vi "2014 Target Detection.vi"() -> (0 "Target Info":T6(array[cluster]))   [LabVIEW 2013]
uses:
  <vilib>/Rock Robotics/WPI/Camera/WPI_CameraSettings Read MJPG.ctl
  <vilib>/Rock Robotics/WPI/Camera/WPI_CameraImageSize.ctl
  TargetType.ctl
  <vilib>/vision/NI_Vision_Development_Module.lvlib
panel:
  out "Angle from Robot (deg)":dbl
  out "Polar Plot":picture
  in  "Instructions:":string="Images:\nUse the tab immediately below to choose the image source. Update the camera settings or the image directory so that you have images or video to test with.\n\nCalibration:\nYou can update Color Component ranges directly, or by clicking and drawing a line on the colored strip in the Image control. The Std Dev multipliers and where the strip is drawn determine the calibration values.\n\nUse Debugging tab to view the result of the color range threshold .\n\nArea Size LImit is used to ignore objects too small or far away to care about.\n\nThe Details tab contains score details for each target and subObject.\n\nCamera Type is used to select lens angles for distance calculation.\n\nVertical strips with no adjacent horizontal strip are identified as \"not hot\" and marked in blue.\nThe numeric scores indicate represent aspect ratio and rectangularity.\n\nWhen both strips are near enough, the pair is identified as \"hot\" and marked in green. Scores\nindicate the left, right, ratio of widths, and vertical positioning.\n\nAny score that falls below cutoff is drawn in red and bounding box is drawn in red."
  in  "Std Devs":cluster{"Hue":dbl, "Sat":dbl, "Val":dbl}={"Hue"=4.0, "Sat"=6.0, "Val"=4.0}
  in  "Area Size Limit %":dbl=0.06 format="%#_13g"
  in  "Camera Type":enum16{"206", "1011", "1013"}(ring)=enum."1013"
  out "loop time ms":u32
  in  "Score Cutoff":dbl(slide)=54.248366013071895 scale=0.0..100.0
  in  "Color Components":T1={"Hue"={80.66666412353516, 112.66666412353516}, "Sat"={0.0, 255.0}, "Val"={102.97300720214844, 167.49366760253906}} {"Val" scale=0.0..255.0; "Sat" scale=0.0..255.0; "Hue" scale=0.0..255.0 scale format="%#_3g"}
  out "Error":bool
  in  "Image Source":enum32{"Files", "Camera"}(tab)=enum."Camera"
  in  "List of image files":i32(listbox)
  in  "Image Directory":path=path "2014 Pseudo-Target/2014 Pseudo-Target Active"
  in  "Camera Settings":T2={"fps"=15, "compression"=5, "Image Size"=enum."640x480"}
  in  "Camera IP":string="10.15.10.11"
  in  "Tabbed Info":enum32{"Debugging", "Details"}(tab)
  out "Mask":T4(plugin-control)
  out "Image":T4(plugin-control)
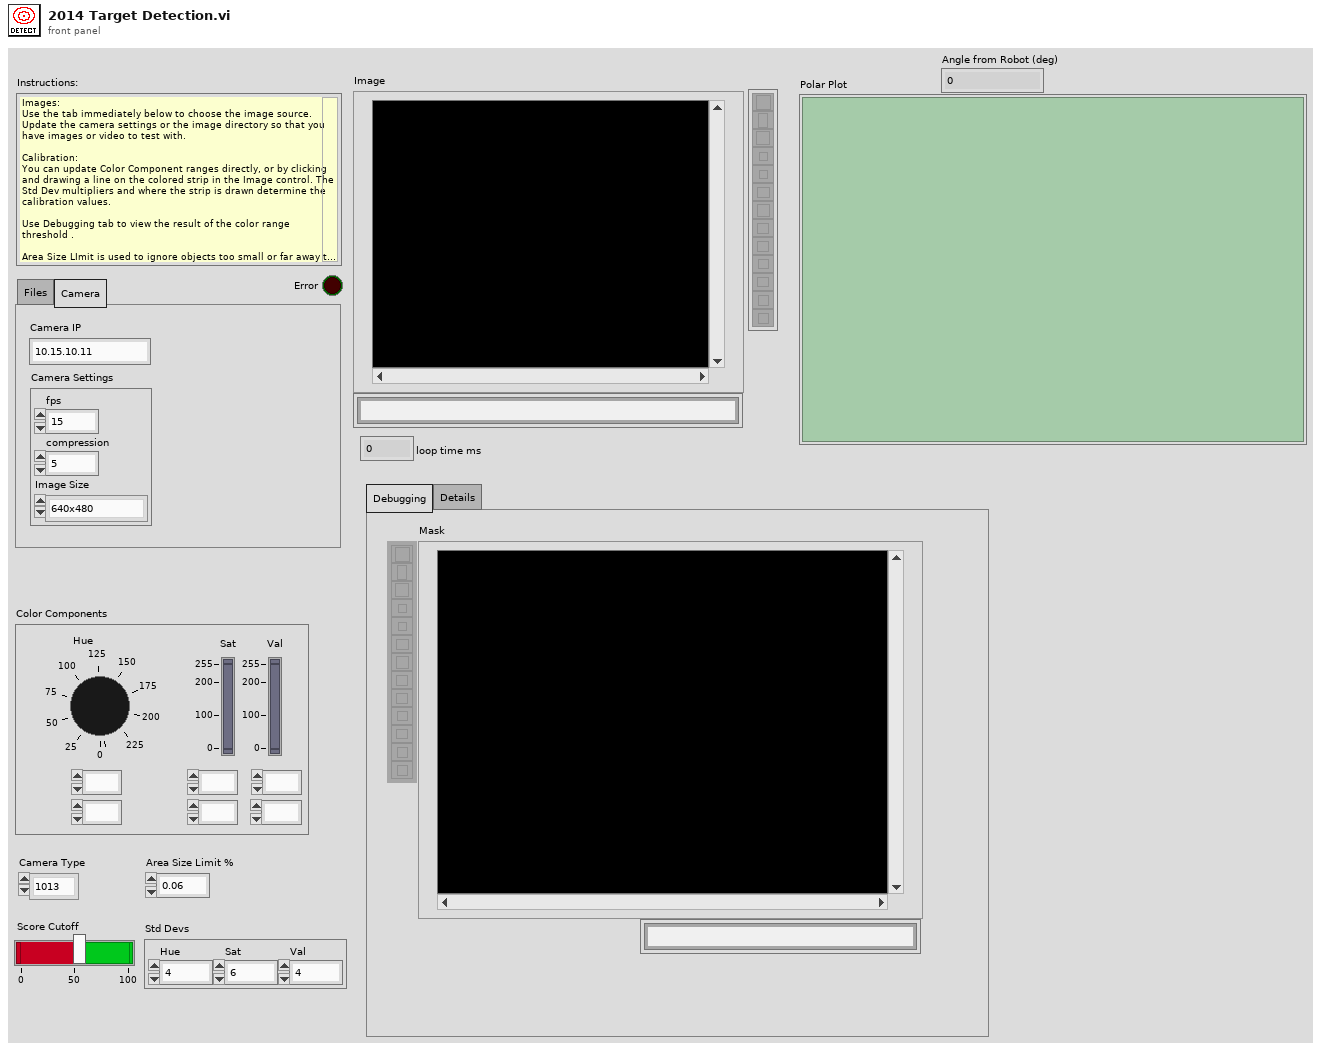
[diagram p1: front panel]
types:
  T1 = cluster{"Hue":cluster{dbl, dbl}, "Sat":cluster{dbl, dbl}, "Val":cluster{dbl, dbl}}
  T2 = typedef "WPI_CameraSettings Read MJPG.ctl" = cluster{"fps":i32, "compression":i32, "Image Size":T3}
  T3 = typedef "WPI_CameraImageSize.ctl" = enum16{"640x480", "320x240", "160x120"}
  T4 = typedef "IMAQ Image.ctl" = refnum<image>
  T5 = typedef "TargetType.ctl" = enum16{"Not Hot", "Hot"}
  T6 = cluster{"Scores":cluster{"Total":dbl, "Left":dbl, "Right":dbl, "Ratio":dbl, "Vertical":dbl, "index":i32, "State":T5}, "Verticals":cluster{"Horizontal?":bool, "Aspect Score":dbl, "Rect Score":dbl, cluster{"Left":dbl, "Top":dbl, "Right":dbl, "Bottom":dbl}, "Equiv H":dbl, "Equiv V":dbl}, "Horizontals":cluster{"Horizontal?":bool, "Aspect Score":dbl, "Rect Score":dbl, cluster{"Left":dbl, "Top":dbl, "Right":dbl, "Bottom":dbl}, "Equiv H":dbl, "Equiv V":dbl}, "Distance ft":dbl, "Center":cluster{"X":dbl, "Y":dbl}}[]
  T7 = typedef "Image Type" = u32
  T8 = cluster{"Horizontal":bool, "Aspect Score":dbl, "Rect Score":dbl, cluster{"Left":dbl, "Top":dbl, "Right":dbl, "Bottom":dbl}, "Equiv H":dbl, "Equiv V":dbl}[]
  T9 = cluster{cluster{dbl, dbl}, cluster{dbl, dbl}, cluster{dbl, dbl}}
  T10 = cluster{"Scores":cluster{"Total":dbl, "Left":dbl, "Right":dbl, "Ratio":dbl, "Vertical":dbl, "index":i32, "State":T5}, "Verticals":cluster{"Horizontal?":bool, "Aspect Score":dbl, "Rect Score":dbl, cluster{"Left":dbl, "Top":dbl, "Right":dbl, "Bottom":dbl}, "Equiv H":dbl, "Equiv V":dbl}, "Horizontals":cluster{"Horizontal?":bool, "Aspect Score":dbl, "Rect Score":dbl, cluster{"Left":dbl, "Top":dbl, "Right":dbl, "Bottom":dbl}, "Equiv H":dbl, "Equiv V":dbl}, "Validated":bool}[]
  T11 = cluster{"Scores":cluster{"Total":dbl, "Left":dbl, "Right":dbl, "Ratio":dbl, "Vertical":dbl, "index":i32, "State":T5}, "Verticals":cluster{"Horizontal?":bool, "Aspect Score":dbl, "Rect Score":dbl, cluster{"Left":dbl, "Top":dbl, "Right":dbl, "Bottom":dbl}, "Equiv H":dbl, "Equiv V":dbl}, "Horizontals":cluster{"Horizontal?":bool, "Aspect Score":dbl, "Rect Score":dbl, cluster{"Left":dbl, "Top":dbl, "Right":dbl, "Bottom":dbl}, "Equiv H":dbl, "Equiv V":dbl}, "Distance (ft)":dbl, "Target Center (-1 to 1)":cluster{"X":dbl, "Y":dbl}}[]
  T12 = cluster{"Scores":cluster{"Total":dbl, "Left":dbl, "Right":dbl, "Ratio":dbl, "Vertical":dbl, "index":i32, "State":T5}, "Verticals":cluster{"Horizontal?":bool, "Aspect Score":dbl, "Rect Score":dbl, cluster{"Left":dbl, "Top":dbl, "Right":dbl, "Bottom":dbl}, "Equiv H":dbl, "Equiv V":dbl}, "Horizontals":cluster{"Horizontal?":bool, "Aspect Score":dbl, "Rect Score":dbl, cluster{"Left":dbl, "Top":dbl, "Right":dbl, "Bottom":dbl}, "Equiv H":dbl, "Equiv V":dbl}, "Distance (ft)":dbl, "Target Center (-1 to 1)":cluster{"X":dbl, "Y":dbl}}
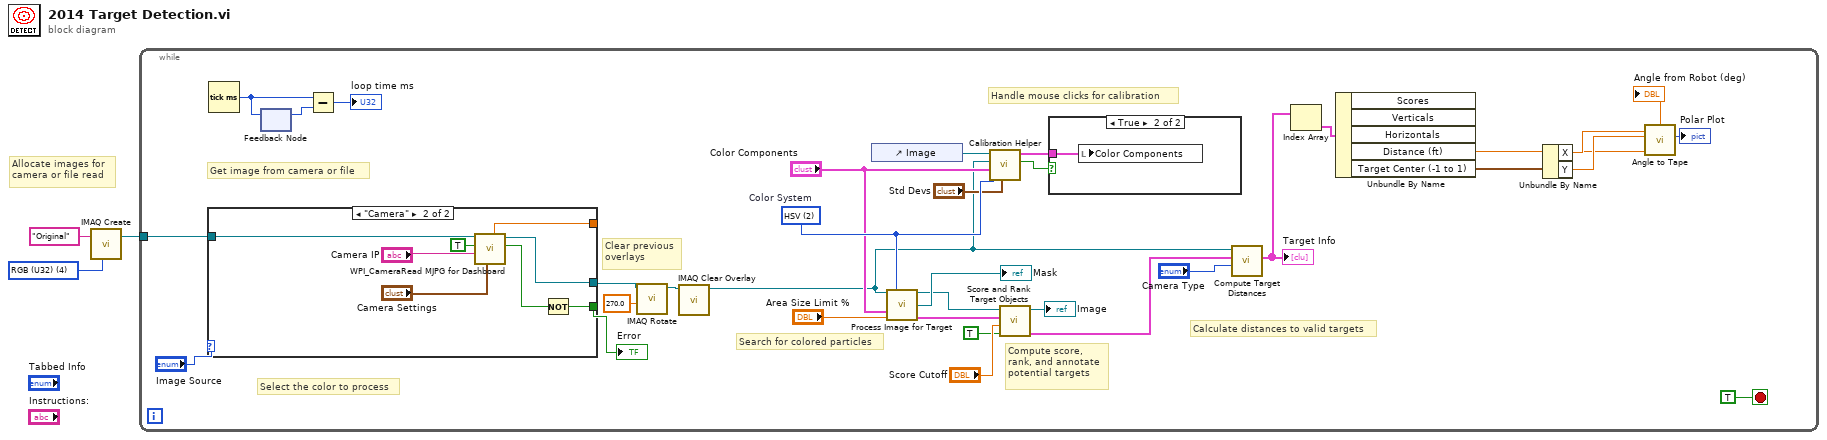
[diagram p0: block diagram]
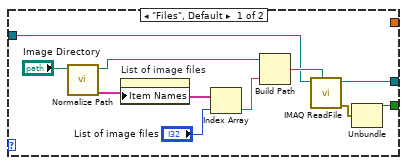
[diagram p3: hidden frame]
diagram:
  w3 = T7 4 items=["Grayscale (U8)", "Grayscale (I16)", "Grayscale (SGL)", "Complex (CSG)", "RGB (U32)", "HSL (U32)", "RGB (U64)", "Grayscale (U16)"] ("Image Type")
  # "Allocate images for\ncamera or file read"
  n1 = call "IMAQ Create"("Image Name"="Original", "Image Type"=w3) -> ("New Image"=w1:T4)  [unwired: 3 in, 1 out]
  n2 = while {
    tunnel: w1 -> [w35]
    stop <- TRUE stop-if-true
    w21 = u16 2 items=["RGB", "HSL", "HSV", "HSI"]  # Color System
    # "Clear previous\noverlays"
    # "Calculate distances to valid targets"
    # "Search for colored particles"
    # "Handle mouse clicks for calibration"
    # "Compute score,\nrank, and annotate\npotential targets"
    # "Select the color to process"
    # "Get image from camera or file"
    n3 = case shown="\"Camera\"" "Image Source" {
      tunnel: [w45 w55] -> w6
      tunnel: w35 -> [w44 w56]
      tunnel: [w42 w50] -> w34
      tunnel: [_ w49] -> _
      frame "Files", Default {
        n4 = call "Normalize Path.vi"("Image Directory"="Image Directory") -> ("Filenames"=w40:string[], "Path"=w39:path)  [unwired: 9 in]
        n5 = property on="List of image files" class="LstBox (strict)"("Item Names"=w40) -> ()  [unwired: 2 in, 2 out]
        n6 = Index Array(array=w40, index="List of image files") -> (element=w47:string)
        n7 = Build Path(base path=w39, name or relative path=w47) -> (appended path=w46:path)
        n8 = call "IMAQ ReadFile"("File Path"=w46, "Image"=w44) -> ("error out"=w43:errorcluster, "Image Out"=w45:T4)  [unwired: 5 in, 3 out]
        n9 = Unbundle(w43) -> ("status"=w42:bool)  [unwired: 2 out]
      }
      frame "Camera" {
        n10 = call <vilib>:"WPI_CameraRead MJPG for Dashboard.vi"("Camera Settings"="Camera Settings", "Camera IP"="Camera IP", "Enable"=TRUE, "Refnum in"=w56) -> ("Active"=w52:bool, "Refnum out"=w55:T4, "Bandwidth (Mbps)"=w49:dbl)  [unwired: 4 in, 1 out]
        n11 = Not(x=w52) -> (.not. x?=w50:bool)
      }
    }
    "Error" <- w34
    n12 = Tick Count (ms)() -> (millisecond timer value=w33:u32)
    n13 = feedback #1() -> (w32:u32)  [unwired: 1 in]
    n14 = feedback-in #1(w33) -> ()
    n15 = Subtract(x=w33, y=w32) -> (x-y=→"loop time ms":u32)
    n16 = call "IMAQ Rotate"("Angle (degrees)"=sgl 270.0, "Image Src"=w6) -> ("Image Dst Out"=w5:T4)  [unwired: 8 in, 1 out]
    n17 = call "IMAQ Clear Overlay"("Image"=w5) -> ("Image Out"=w16:T4)  [unwired: 9 in, 1 out]
    n18 = control-ref of="Image"() -> (w22:refnum<vi>)
    n19 = call "Process Image for Target.vi"("Src Image"=w16, "Color Mode"=w21, "Color Components"="Color Components", "Area Cutoff %"="Area Size Limit %") -> ("Src Image Out"=w28:T4, "Threshold"=→"Mask":T4, "Particles"=w25:T8)  [unwired: 9 in]
    n20 = call "Calibration Helper.vi"("Std Devs"="Std Devs", "Color Mode"=w21, "Color Components"="Color Components", "Image"=w16, "Image Ctl Refnum"=w22) -> ("Changed"=w17:bool, "output color"=w19:T9)  [unwired: 5 in]
    n21 = call "Score and Rank Target Objects.vi"("Annotate"=TRUE, "Score Limit"="Score Cutoff", "Particles"=w25, "Image in"=w28) -> ("Target Info"=w24:T10, "Annotated Image"=→"Image":T4)  [unwired: 6 in]
    n22 = case shown="True" w17 {
      tunnel: w19 -> [_ w38]
      frame False {
      }
      frame True {
        n23 = local write "Color Components"(w38) -> ()
      }
    }
    n24 = call "Compute Target Distances.vi"("Camera Type"="Camera Type", "Target Info"=w24, "Image in"=w16) -> ("Target Info"=w14:T11)  [unwired: 6 in, 2 out]
    "Target Info" <- w14
    n25 = Index Array(array=w14) -> (element=w13:T12)  [unwired: 1 in]
    n26 = Unbundle By Name(w13) -> ("Distance (ft)"=w9:dbl, "Target Center (-1 to 1)"=w12:cluster{"X":dbl, "Y":dbl})  [unwired: 3 out]
    n27 = Unbundle By Name(w12) -> ("X"=w11:dbl, "Y"=w10:dbl)
    n28 = call "Angle to Tape.vi"("Distance To Target (ft)"=w9, "Y"=w10, "X"=w11) -> ("Polar Plot"=→"Polar Plot":picture, "Angle from Robot (deg)"=→"Angle from Robot (deg)":dbl)  [unwired: 7 in]
  }
